vi "Runtime Configuration Support Inline Async Example Custom Device.Async.vi"(10 "Parameters":variant, 11 "Process":refnum<class "Process.lvclass">) -> ()   [LabVIEW 2026, in "Runtime Configuration Support Inline Async Example Custom Device Engine.lvlib"]
uses:
  Runtime Configuration Support Inline Async Example Custom Device Engine.lvlib
  <vilib>/NI/NIVS Inline Async API/_VS Inline Async API/Process/Process.lvclass
  Parameter.ctl
  Shared/Compiled.Settings.ctl
  AsyncRequest.ctl
  <vilib>/NI/NIVS Inline Async API/_VS Inline Async API/Process/Process.lvclass/Process.ctl
  <vilib>/NI/NIVS Inline Async API/_Data Access Engine/Access Type Classes/Read/Read.lvclass/Read.ctl
  <vilib>/NI/NIVS Inline Async API/_Data Access Engine/Access Type Classes/Write/Write.lvclass/Write.ctl
  <vilib>/NI/NIVS Inline Async API/_Data Access Engine/Data Access Engine/Methods/Write.Data.vi
  <vilib>/NI/NIVS Inline Async API/_VS Inline Async API/Process/Data Member Access/Read Data Access.vi
  <vilib>/NI/NIVS Inline Async API/_VS Inline Async API/Error Handling Process/SubVIs/Error.ConvertArray.vi
  <vilib>/NI/NIVS Inline Async API/_Data Access Engine/Access Type Classes/Write/Write.ProcessData.vi
  <vilib>/NI/NIVS Inline Async API/_Data Access Engine/Access Type Classes/Read/Read.ProcessData.vi
  <vilib>/NI/NIVS Inline Async API/_Data Access Engine/Access Type Classes/Write/Write.Buffer.vi
  <vilib>/NI/NIVS Inline Async API/_Data Access Engine/Access Type Classes/Write/Write.Commit.vi
  <vilib>/NI/NIVS Inline Async API/_Data Access Engine/Data Access Engine/Methods/Write.Lookup.vi
  <vilib>/NI/NIVS Inline Async API/_Data Access Engine/Data Access Engine/Data Access Engine.lvclass
  Shared/Runtime Configuration Support Inline Async Example Custom Device Shared.lvlib
  <vilib>/NI/NIVS Inline Async API/_Data Access Engine/Data Access Engine/Methods/ReadWrite.Lookup.vi
  <vilib>/NI/NIVS Inline Async API/_Data Access Engine/Data Access Engine/Methods/ReadWrite.Data.Read.vi
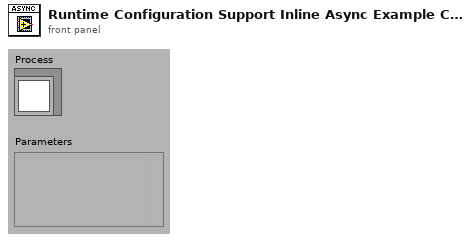
[diagram p1: front panel]
types:
  T1 = typedef "Runtime Configuration Support Inline Async Example Custom Device Engine.lvlib/Parameter.ctl" = cluster{"Compiled.Settings":T2, "Async Request Ref":refnum<queue>}
  T2 = typedef "Runtime Configuration Support Inline Async Example Custom Device Shared.lvlib/Compiled.Settings.ctl" = cluster{"Name":string, "Async Init Timeout":u16, "Inport SignalIDs":i32[], "Outport SignalIDs":i32[], "Inport Values":dbl[], "Outport Values":dbl[], "Dynamic Config Status":bool, "Device Error":errorcluster}
  T3 = enum16{"Initialize", "Set In Val", "Get In Val", "Set Block", "Set Out Val", "Get Out Val", "Get In Array", "Get Out Array"}
  T4 = typedef "Data Access Engine.lvlib/Data Access Engine.lvclass/Write.DVR.ctl" = refnum<data-value>
  T5 = typedef "Data Access Engine.lvlib/Data Access Engine.lvclass/ReadWrite.DVR.ctl" = refnum<data-value>
  T6 = typedef "Runtime Configuration Support Inline Async Example Custom Device Engine.lvlib/AsyncRequest.ctl" = cluster{"Compiled.Settings":T2, "Data Access":variant, "Async Response Ref":refnum<queue>}
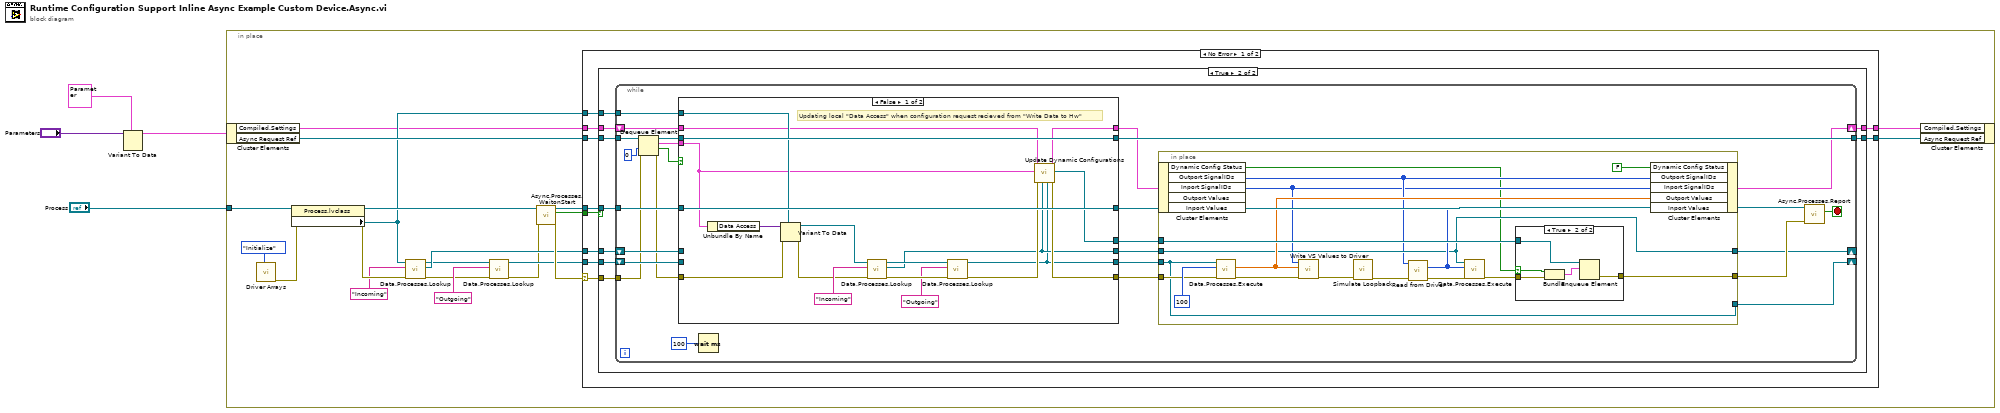
[diagram p0: block diagram]
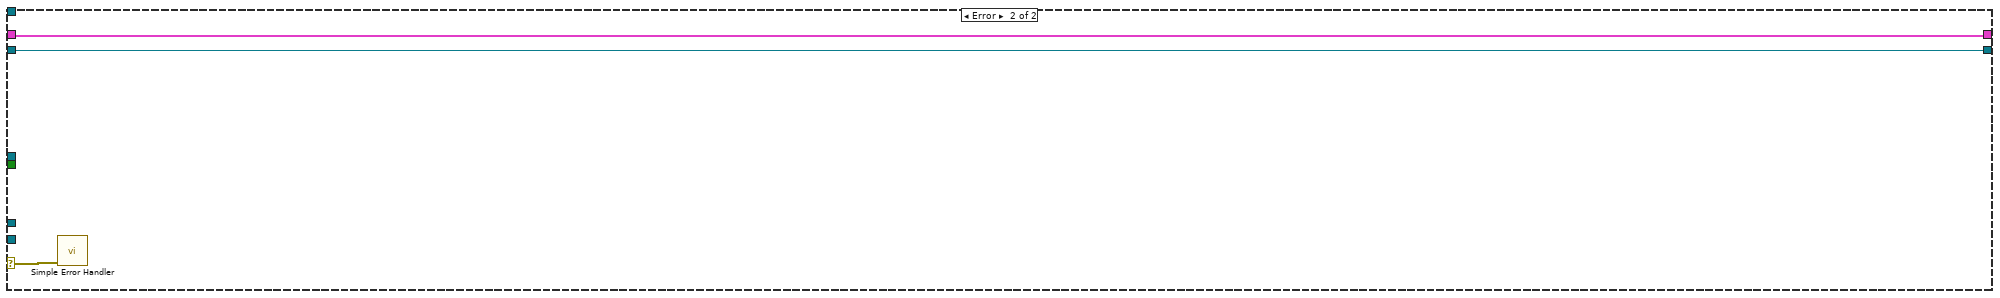
[diagram p5: hidden frame]
diagram:
  n1 = Variant To Data(type=T1 {"Compiled.Settings"={"Name"="", "Async Init Timeout"=0, "Inport SignalIDs"=[], "Outport SignalIDs"=[], "Inport Values"=[], "Outport Values"=[], "Dynamic Config Status"=FALSE, "Device Error"={"status"=FALSE, "code"=0, "source"=""}}, "Async Request Ref"=refnum} ("Parameter"), Variant="Parameters") -> (data=w2:T1)  [unwired: 1 in, 1 out]
  n2 = in-place {
    in-place-border: "Process" -> [w16]
    n3 = in-place-cluster #1(w2) -> ("Compiled.Settings"=w8:T2, "Async Request Ref"=w15:refnum<queue>)
    n4 = call "Driver Arrays.vi"("Curr Operation"=T3."Initialize") -> ("error out"=w6:errorcluster)  [unwired: 7 in, 3 out]
    n5 = property class="Process.lvclass"(reference=w16, error in=w6) -> (reference out=w18:refnum<class "Process.lvclass">, error out=w17:errorcluster, "Data Member Access:Data Access"=w14:refnum<class "Data Access Engine.lvclass">)
    n6 = call-poly <vilib>:"Data.Processes.Lookup.vi"("error in (no error)"=w17, "Name"="Incoming", "Data Access API in"=w14) -> ("error out"=w10:errorcluster, "Ref"=w20:T4, "Data Access API out"=w9:refnum<class "Data Access Engine.lvclass">)  [unwired: 5 in, 1 out]
    n7 = call-poly <vilib>:"Data.Processes.Lookup.vi"("error in (no error)"=w10, "Name"="Outgoing", "Data Access API in"=w9) -> ("error out"=w19:errorcluster, "Ref"=w21:T5)  [unwired: 5 in, 2 out]
    n8 = call <vilib>:"Async.Processes.WaitonStart.vi"("error in (no error)"=w19, "Process"=w18) -> ("error out"=w22:errorcluster, "Execute"=w24:bool, "Process out"=w23:refnum<class "Process.lvclass">)  [unwired: 7 in]
    n9 = case shown="No Error" w22 {
      selector: w22 -> [w30 w121]
      tunnel: w24 -> [w34 _]
      tunnel: w23 -> [w33 _]
      tunnel: w20 -> [w32 _]
      tunnel: w21 -> [w31 _]
      tunnel: w15 -> [w29 w120]
      tunnel: w14 -> [w28 _]
      tunnel: [w27 w120] -> w13
      tunnel: w8 -> [w26 w119]
      tunnel: [w25 w119] -> w7
      frame No Error {
        n10 = case shown="True" w34 {
          tunnel: w30 -> [_ w42]
          tunnel: w33 -> [_ w43]
          tunnel: w31 -> [_ w45]
          tunnel: w32 -> [_ w44]
          tunnel: w29 -> [w36 w41]
          tunnel: w28 -> [_ w40]
          tunnel: [w36 w39] -> w27
          tunnel: w26 -> [w35 w38]
          tunnel: [w35 w37] -> w25
          frame False {
          }
          frame True {
            n11 = while {
              tunnel: w42 -> [w55]
              tunnel: w43 -> [w68]
              tunnel: w41 -> [w58]
              tunnel: w40 -> [w61]
              tunnel: [w59] -> w39
              shift-right: [w48] -> _
              shift-left: w44 -> [w65]
              shift-right: [w47] -> _
              shift-left: w45 -> [w64]
              shift-right: [w49] -> w37
              shift-left: w38 -> [w53]
              stop <- w70 stop-if-true
              n12 = Dequeue Element(queue=w58, timeout in ms (-1)=0, error in (no error)=w55) -> (queue out=w60:refnum<queue>, element=w62:T6, timed out?=w66:bool, error out=w54:errorcluster)
              n13 = case shown="False" w66 {
                tunnel: w68 -> [w112 w118]
                tunnel: [w112 w118] -> w67
                tunnel: w65 -> [_ w117]
                tunnel: [w95 w117] -> w57
                tunnel: w64 -> [_ w116]
                tunnel: [w94 w116] -> w56
                tunnel: w54 -> [w103 w115]
                tunnel: [w96 w115] -> w63
                tunnel: w62 -> [w100 _]
                tunnel: w61 -> [w105 _]
                tunnel: w60 -> [w111 w114]
                tunnel: [w111 w114] -> w59
                tunnel: w53 -> [w101 w113]
                tunnel: [w99 w113] -> w50
                tunnel: [w98 _] -> w52
                frame False {
                  # "Updating local \"Data Access\" when configuration request recieved from \"Write Data to Hw\""
                  n14 = Unbundle By Name(w100) -> ("Data Access"=w106:variant)
                  n15 = Variant To Data(error in=w103, type=w105, Variant=w106) -> (data=w104:refnum<class "Data Access Engine.lvclass">, error out=w102:errorcluster)
                  n16 = call-poly <vilib>:"Data.Processes.Lookup.vi"("error in (no error)"=w102, "Name"="Incoming", "Data Access API in"=w104) -> ("error out"=w109:errorcluster, "Ref"=w95:T4, "Data Access API out"=w110:refnum<class "Data Access Engine.lvclass">)  [unwired: 5 in, 1 out]
                  n17 = call-poly <vilib>:"Data.Processes.Lookup.vi"("error in (no error)"=w109, "Name"="Outgoing", "Data Access API in"=w110) -> ("error out"=w97:errorcluster, "Ref"=w94:T5)  [unwired: 5 in, 2 out]
                  n18 = call "Update Dynamic Configurations.vi"("Write Ref"=w95, "Read Write Ref"=w94, "error in"=w97, "AsyncRequest"=w100, "Compiled.Settings in"=w101) -> ("error out"=w96:errorcluster, "Response Ref"=w98:refnum<queue>, "Compiled.Settings out"=w99:T2)  [unwired: 4 in]
                }
                frame True {
                }
              }
              n19 = Wait (ms)(milliseconds to wait=u32 100) -> ()  [unwired: 1 out]
              n20 = in-place {
                in-place-border: w63 -> [w86]
                in-place-border: w57 -> [w75]
                in-place-border: w56 -> [w71]
                in-place-border: w52 -> [w81]
                in-place-border: [w76] -> w51
                in-place-border: [w75] -> w48
                in-place-border: [w71] -> w47
                n21 = in-place-cluster #2(w50) -> ("Dynamic Config Status"=w72:bool, "Outport SignalIDs"=w74:i32[], "Inport SignalIDs"=w73:i32[])  [unwired: 2 out]
                n22 = call-poly <vilib>:"Data.Processes.Execute.vi"("error in (no error)"=w86, "timeout ms"=100, "Ref"=w71) -> ("error out"=w85:errorcluster, "Data"=w78:dbl[])  [unwired: 5 in, 2 out]
                n23 = call "Write VS Values to Driver.vi"("error in"=w85, "VS Values"=w78, "Signal Indices In"=w73) -> ("error out"=w84:errorcluster)  [unwired: 8 in]
                n24 = call "Simulate Loopback.vi"("error in"=w84) -> ("error out"=w83:errorcluster)  [unwired: 10 in]
                n25 = call "Read from Driver.vi"("error in"=w83, "Signal Indices Out"=w74) -> ("error out"=w82:errorcluster, "Driver Values"=w77:i32[])  [unwired: 8 in]
                n26 = call-poly <vilib>:"Data.Processes.Execute.vi"("error in (no error)"=w82, "Values"=w77, "Ref"=w75) -> ("error out"=w80:errorcluster)  [unwired: 8 in]
                n27 = case shown="True" w72 {
                  selector: w72 -> [_ w92]
                  tunnel: w81 -> [_ w93]
                  tunnel: w80 -> [w88 w91]
                  tunnel: [w88 w89] -> w76
                  frame False {
                  }
                  frame True {
                    n28 = Bundle(w92, "error out"=w91) -> (w90:cluster{bool, "error out":errorcluster})  [unwired: 1 in]
                    n29 = Enqueue Element(queue=w93, element=w90) -> (error out=w89:errorcluster)  [unwired: 2 in, 2 out]
                  }
                }
                n30 = in-place-cluster #2("Dynamic Config Status"=FALSE, "Outport SignalIDs"=w74, "Inport SignalIDs"=w73, "Outport Values"=w78, "Inport Values"=w77) -> (w49:T2)
              }
              n31 = call <vilib>:"Async.Processes.Report.vi"("Error"=w51, "Process in"=w67) -> ("Stop"=w70:bool)  [unwired: 8 in, 1 out]
            }
          }
        }
      }
      frame Error {
        n32 = call <vilib>:"Simple Error Handler.vi"("error in (no error)"=w121) -> ()  [unwired: 4 in, 5 out]
      }
    }
    n33 = in-place-cluster #1("Compiled.Settings"=w7, "Async Request Ref"=w13) -> ()  [unwired: 1 out]
  }
